vi "Build Report String.vi"(8 "error in (no error)":errorcluster, 10 "Report Data":T1, 11 "Numeric Assertion in":refnum<class "Numeric Assertion.lvclass">) -> (0 "error out":errorcluster, 2 "Report String":string, 3 "Numeric Assertion out":refnum<class "Numeric Assertion.lvclass">)   [LabVIEW 2020, in "MacroAssert.lvlib" / "Numeric Assertion.lvclass"]
doc: "Builds a string using <B>Step</B> and <B>Report Data</B> to be included in a report."
uses:
  Numeric Assertion.lvclass
  Numeric Assertion.lvclass/Numeric Assertion.ctl
  CTLs/Report Data.ctl
  MacroAssert.lvlib
  CTLs/Result.ctl
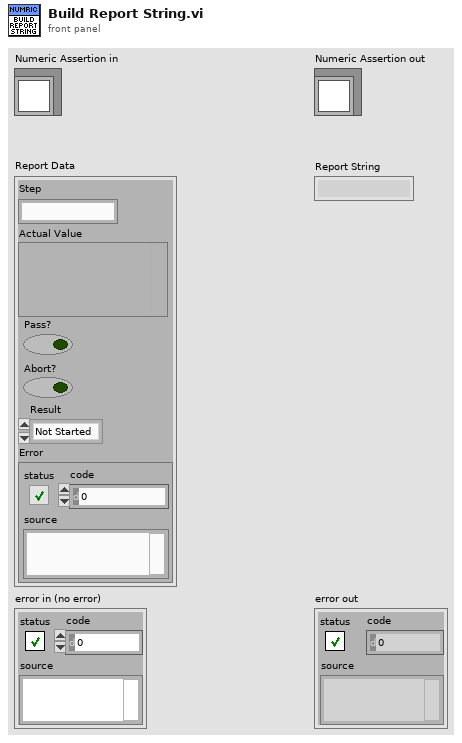
[diagram p1: front panel]
types:
  T1 = typedef "MacroAssert.lvlib/Report Data.ctl" = cluster{"Step":string, "Actual Value":variant, "Pass?":bool, "Abort?":bool, "Result":T2, "Error":errorcluster}
  T2 = typedef "MacroAssert.lvlib/Result.ctl" = enum16{"Not Started", "Skipped", "Pass", "Fail", "Complete", "Error"}
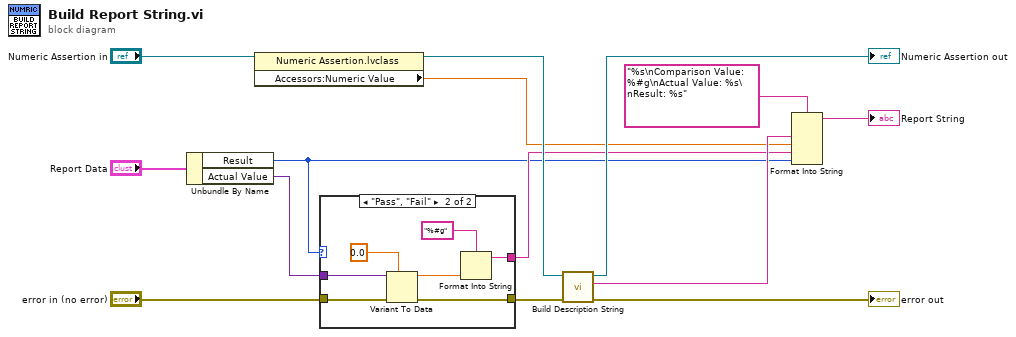
[diagram p0: block diagram]
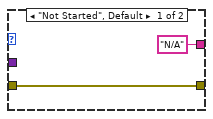
[diagram p2: hidden frame]
diagram:
  n1 = Unbundle By Name("Report Data") -> ("Result"=w1:T2, "Actual Value"=w5:variant)
  n2 = property class="Numeric Assertion.lvclass"(reference="Numeric Assertion in") -> (reference out=w4:refnum<class "Numeric Assertion.lvclass">, "Accessors:Numeric Value"=w3:dbl)  [unwired: 1 in, 1 out]
  n3 = case shown="\"Pass\", \"Fail\"" w1 {
    tunnel: "error in (no error)" -> [w16 w23]
    tunnel: [w16 w22] -> w6
    tunnel: w5 -> [_ w21]
    tunnel: ["N/A" w17] -> w2
    frame "Not Started", Default {
    }
    frame "Pass", "Fail" {
      n4 = Variant To Data(error in=w23, type=0.0, Variant=w21) -> (data=w18:dbl, error out=w22:errorcluster)
      n5 = Format Into String(format string="%#g", w18) -> (resulting string=w17:string)  [unwired: 2 in, 1 out]
    }
  }
  n6 = call-dynamic "Build Description String.vi"("error in (no error)"=w6, "Numeric Assertion in"=w4) -> ("error out"=→"error out":errorcluster, "Description"=w13:string, "Numeric Assertion out"=→"Numeric Assertion out":refnum<class "Numeric Assertion.lvclass">)  [unwired: 7 in]
  n7 = Format Into String(format string="%s\nComparison Value: %#g\nActual Value: %s\nResult: %s", w13, w3, w2, w1) -> (resulting string=→"Report String":string)  [unwired: 2 in, 1 out]
